vi "Licor data processing.vi"(8 "command parameter":T2={"CO2 ref"=392.0, "CO2 span"=372.0, "H2O ref"=0.0, "H2O span"=0.0, "Zi"=0.0, "Zt"=1.2, "Zm"=0.0, "S"=0.0, "Temp [C]"=50.0, "Pressure [hPa]"=135.0, "Licor-Sources"=["CO2A W", "CO2B W", "H2OA W", "H2OB W", "T C", "T V", "P kPa", "P V", "RH %", "CO2A um/m", "CO2B um/m", "H2OA mm/m", "H2OB mm/m"], "Licor-Pump"="Off", "Zeitstempel"=timestamp(0 s since 1904-01-01)} {"Pressure [hPa]" format="%_5g"; "Temp [C]" format="%.2f"; "CO2 ref" format="%.2f"; "CO2 span" format="%.2g"; "H2O ref" format="%.2g"; "H2O span" format="%.2g"; "Zt" format="%#_4g"}, 9 "mittel CO2B W":dbl[](array[numeric]), 10 "mittel CO2A W":dbl[](array[numeric]), 11 "data":T1[](array[typedef]) {"time (global)" format="%<%H:%M:%S\n%d/%m/%Y>T"}) -> (0 "time; CO2 data":dbl[][](array[numeric]), 1 "mittel CO2B W out":dbl[](array[numeric]), 2 "mittel CO2A W out":dbl[](array[numeric]), 3 "command parameter":T2={"CO2 ref"=0.0, "CO2 span"=0.0, "H2O ref"=0.0, "H2O span"=0.0, "Zi"=0.0, "Zt"=0.0, "Zm"=0.0, "S"=0.0, "Temp [C]"=50.0, "Pressure [hPa]"=135.0, "Licor-Sources"=["CO2A W", "CO2B W", "H2OA W", "H2OB W", "T C", "T V", "P kPa", "P V", "RH %", "CO2A um/m", "CO2B um/m", "H2OA mm/m", "H2OB mm/m"], "Licor-Pump"="Off", "Zeitstempel"=timestamp(0 s since 1904-01-01)} {"Pressure [hPa]" format="%_5g"; "Temp [C]" format="%.2f"; "CO2 ref" format="%.2f"; "CO2 span" format="%.2g"; "H2O ref" format="%.2g"; "H2O span" format="%.2g"; "Zt" format="%#_4g"})   [LabVIEW 2017, in "Licor-Steuerung.lvlib"]
uses:
  Licor-Steuerung.lvlib
  control/Licor-Parameter.ctl
  LicorLI7000/conventions/Licor-Source.ctl
  control/Licor-Pump.ctl
  LicorLI7000/conventions/output line.ctl
  LicorLI7000/Z parameter.ctl
  LicorLI7000/LicorLI7000.lvlib
panel:
  in  "get Source":string(combo)="CO2A W"
  out "calibration data out":dbl[][](array[numeric])
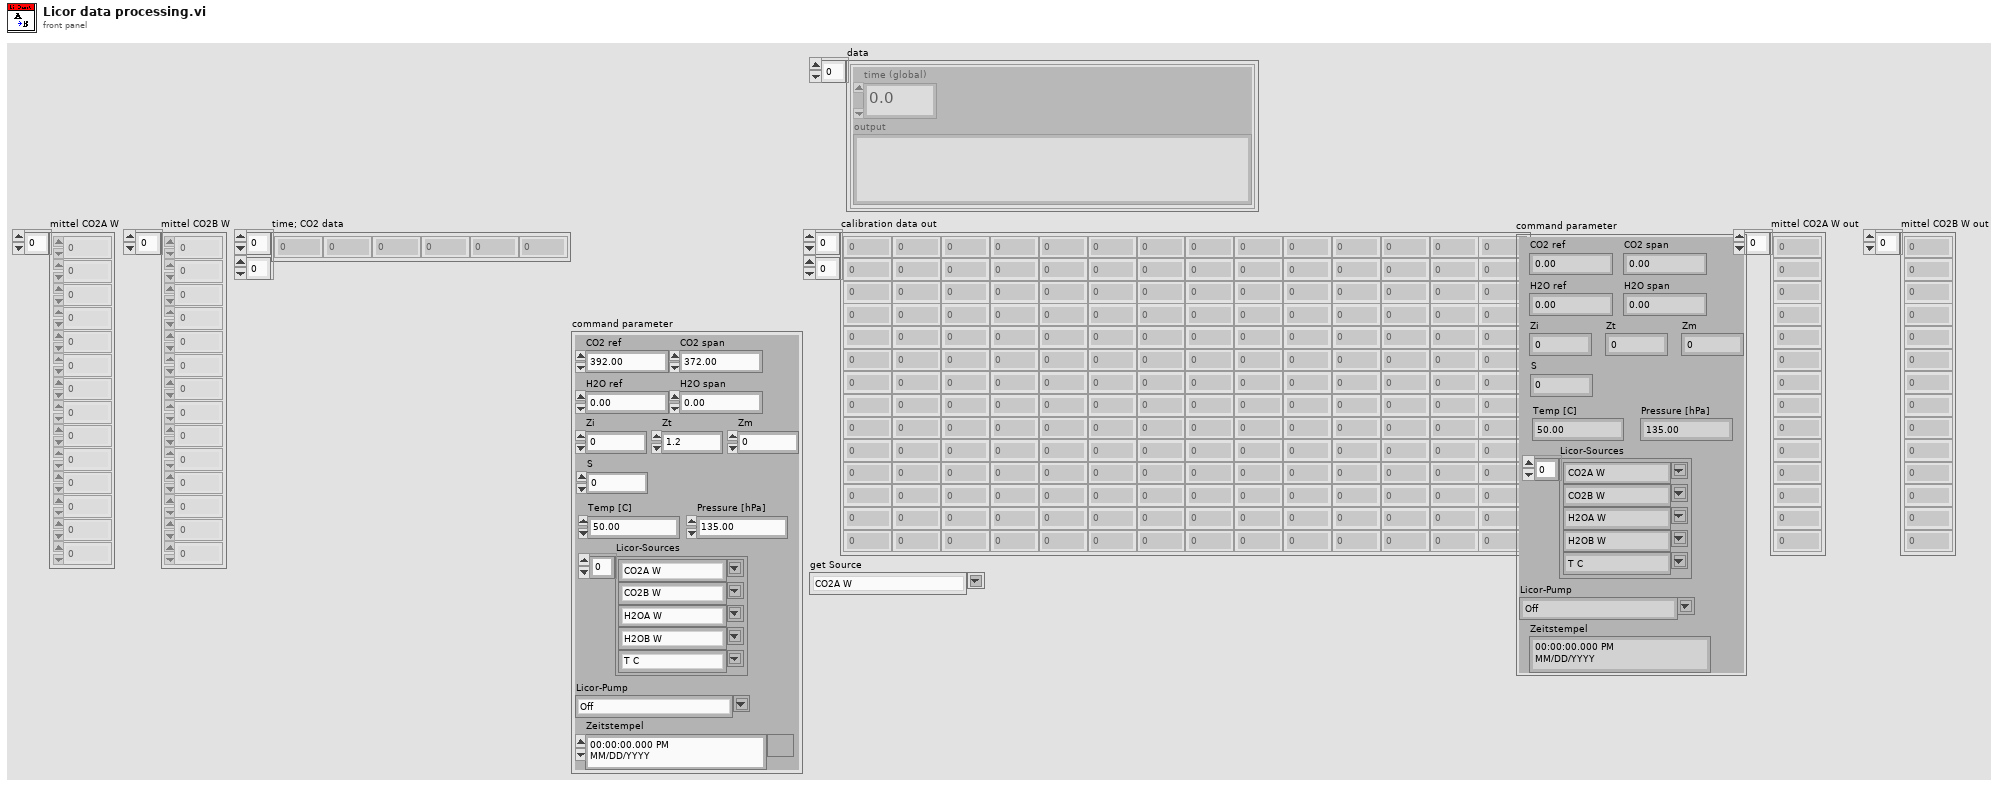
[diagram p1: front panel]
types:
  T1 = typedef "LicorLI7000.lvlib/output line.ctl" = cluster{"time (global)":dbl, "output":string}
  T2 = typedef "Licor-Steuerung.lvlib/Licor-Parameter.ctl" = cluster{"CO2 ref":dbl, "CO2 span":dbl, "H2O ref":dbl, "H2O span":dbl, "Zi":dbl, "Zt":dbl, "Zm":dbl, "S":dbl, "Temp [C]":dbl, "Pressure [hPa]":dbl, "Licor-Sources":T3[], "Licor-Pump":T4, "Zeitstempel":timestamp}
  T3 = typedef "LicorLI7000.lvlib/Licor-Source.ctl" = string
  T4 = typedef "Licor-Steuerung.lvlib/Licor-Pump.ctl" = string
  T5 = typedef "LicorLI7000.lvlib/Z parameter.ctl" = cluster{"zi":dbl, "zt":dbl, "zm":dbl}
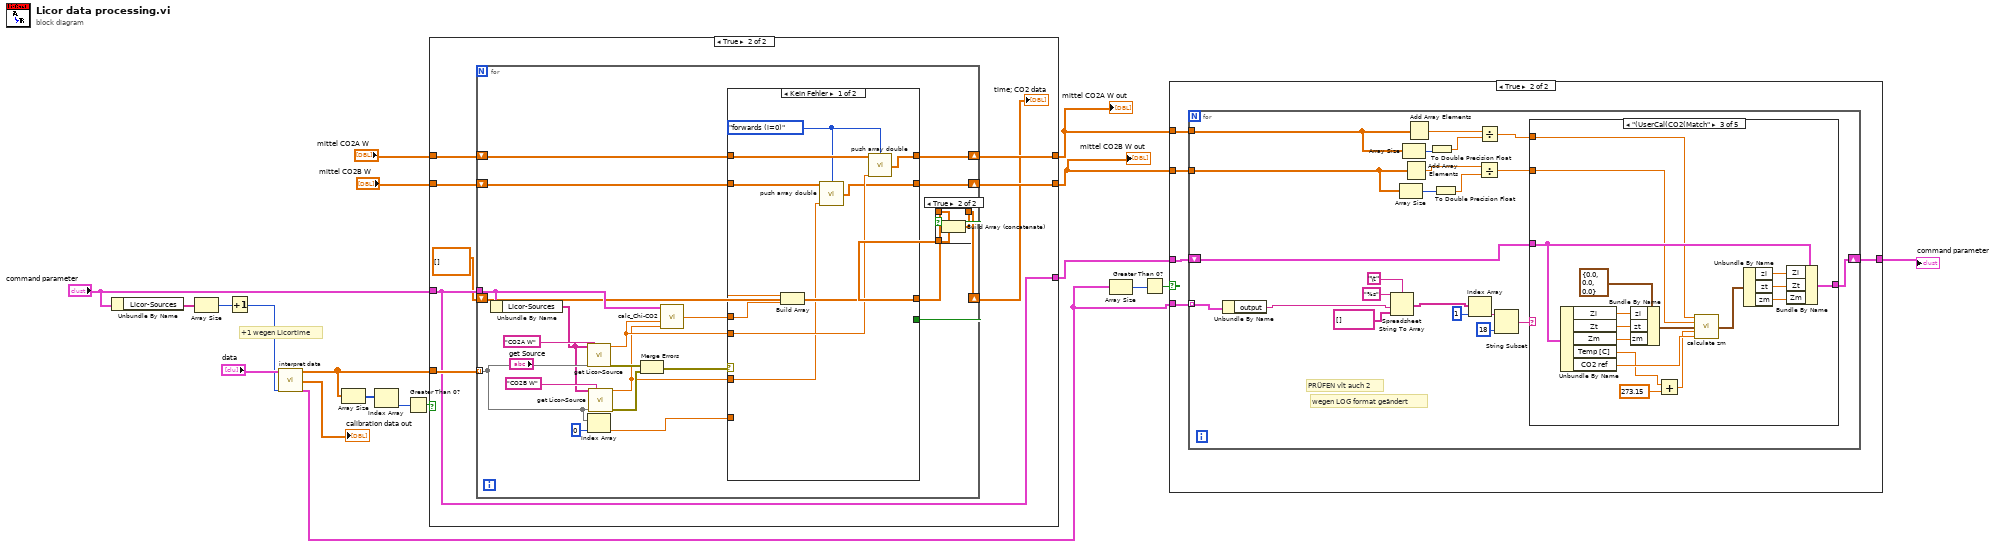
[diagram p0: block diagram]
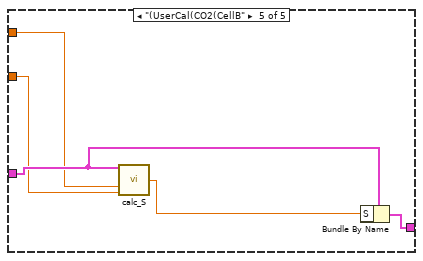
[diagram p6: hidden frame]
diagram:
  # "+1 wegen Licortime"
  n1 = Unbundle By Name("command parameter") -> ("Licor-Sources"=w4:T3[])
  n2 = Array Size(array=w4) -> (size(s)=w3:i32)
  n3 = Increment(x=w3) -> (x+1=w2:i32)
  n4 = call "interpret data.vi"("data"="data", "anzahl sources"=w2) -> ("source data out"=w18:dbl[][], "calibration data out"=→"calibration data out":dbl[][], "log"=w1:T1[])  [unwired: 11 in]
  n5 = Array Size(array=w18) -> (size(s)=w17:i32[])
  n6 = Index Array(array=w17) -> (element=w16:i32)  [unwired: 1 in]
  n7 = Greater Than 0?(x=w16) -> (x > 0?=w19:bool)
  n8 = case shown="True" w19 {
    tunnel: w18 -> [_ w30]
    tunnel: "command parameter" -> [w22 w29]
    tunnel: [w22 w29] -> w14
    tunnel: "mittel CO2A W" -> [w21 w28]
    tunnel: "mittel CO2B W" -> [w20 w27]
    tunnel: [w21 w26] -> w10
    tunnel: [w20 w25] -> w9
    frame False {
    }
    frame True {
      n9 = for {
        tunnel: w30 -> [w38] mode=indexing
        tunnel: w29 -> [w34]
        shift-right: [w41] -> w26
        shift-left: w28 -> [w43]
        shift-right: [w40] -> w25
        shift-left: w27 -> [w42]
        shift-right: [w31] -> w24
        shift-left: dbl[][] [] ("Array") -> [w32]
        n10 = Unbundle By Name(w34) -> ("Licor-Sources"=w33:T3[])
        n11 = call "get Licor-Source.vi"("Sources"=w33, "get Source"="CO2A W", "source data"=w38) -> ("value"=w45:dbl, "Fehlerkonstante"=w48:errorcluster)  [unwired: 10 in, 1 out]
        n12 = Index Array(array=w38, index=0 ("Index")) -> (element=w37:dbl)
        n13 = call "get Licor-Source.vi"("Sources"=w33, "get Source"="CO2B W", "source data"=w38) -> ("value"=w44:dbl, "Fehlerkonstante"=w49:errorcluster)  [unwired: 10 in, 1 out]
        n14 = Merge Errors(w48, w49) -> (w47:errorcluster)
        n15 = call "calc_Chi-CO2.vi"("command parameter"=w34, "Raw_CO2_A"=w45, "Raw_CO2_B"=w44) -> ("Chi_CO2_B"=w46:dbl)  [unwired: 12 in]
        n16 = case shown="Kein Fehler" w47 {
          tunnel: [w57 dbl[] []] -> w36
          tunnel: w46 -> [w66 _]
          tunnel: w44 -> [w59 _]
          tunnel: w45 -> [w64 _]
          tunnel: w43 -> [w65 w70]
          tunnel: w42 -> [w62 w69]
          tunnel: [w63 w70] -> w41
          tunnel: [w60 w69] -> w40
          tunnel: w37 -> [w58 _]
          tunnel: [TRUE FALSE] -> w35
          frame No Error {
            w61 = enum16{"forwards (i=0)", "backwards (i=n)"}."forwards (i=0)" ("mode")
            n17 = Build Array(w58, w66) -> (w57:dbl[])
            n18 = call "push array double.vi"("Array"=w62, "mode"=w61, "Element"=w59) -> ("Array out"=w60:dbl[])  [unwired: 12 in]
            n19 = call "push array double.vi"("Array"=w65, "mode"=w61, "Element"=w64) -> ("Array out"=w63:dbl[])  [unwired: 12 in]
          }
          frame Error {
          }
        }
        n20 = case shown="True" w35 {
          tunnel: w32 -> [w52 w54]
          tunnel: w36 -> [_ w53]
          tunnel: [w52 w55] -> w31
          frame False {
          }
          frame True {
            n21 = Build Array (concatenate)(w54, w53) -> (w55:dbl[][])
          }
        }
      }
      "time; CO2 data" <- w24
    }
  }
  "mittel CO2A W out" <- w10
  "mittel CO2B W out" <- w9
  n22 = Array Size(array=w1) -> (size(s)=w6:i32)
  n23 = Greater Than 0?(x=w6) -> (x > 0?=w13:bool)
  n24 = case shown="True" w13 {
    tunnel: w1 -> [_ w76]
    tunnel: w14 -> [w71 w75]
    tunnel: w9 -> [_ w74]
    tunnel: w10 -> [_ w73]
    tunnel: [w71 w72] -> w8
    frame False {
    }
    frame True {
      n25 = for {
        tunnel: w76 -> [w78] mode=indexing
        shift-right: [w95] -> w72
        shift-left: w75 -> [w83]
        tunnel: w73 -> [w85]
        tunnel: w74 -> [w84]
        # "wegen LOG format geändert"
        # "PRÜFEN vlt auch 2"
        n26 = Unbundle By Name(w78) -> ("output"=w77:string)
        n27 = Spreadsheet String To Array(delimiter (Tab)="\t", format string="%s", spreadsheet string=w77, array type (2D Dbl)=string[] []) -> (array=w79:string[])
        n28 = Array Size(array=w84) -> (size(s)=w92:i32)
        n29 = Array Size(array=w85) -> (size(s)=w91:i32)
        n30 = Add Array Elements(numeric array=w84) -> (sum=w89:dbl)
        n31 = Add Array Elements(numeric array=w85) -> (sum=w93:dbl)
        n32 = To Double Precision Float(number=w91) -> (double precision float=w90:dbl)
        n33 = To Double Precision Float(number=w92) -> (double precision float=w88:dbl)
        n34 = Index Array(array=w79, index=1 ("Index")) -> (element=w96:string)
        n35 = Divide(x=w89, y=w88) -> (x/y=w86:dbl)
        n36 = Divide(x=w93, y=w90) -> (x/y=w87:dbl)
        n37 = String Subset(string=w96, length (rest)=18 ("Länge (Rest)")) -> (substring=w94:string)  [unwired: 1 in]
        n38 = case shown="\"(UserCal(CO2(Match\"" w94 {
          tunnel: w83 -> [w99 w100 w115 w118 w123]
          tunnel: [w99 w100 w117 w118 w122] -> w95
          tunnel: w87 -> [_ _ w110 _ w120]
          tunnel: w86 -> [_ _ w109 _ w119]
          frame "False", Default {
          }
          frame "(UserCal(H2O(Match" {
          }
          frame "(UserCal(CO2(Match" {
            n39 = Unbundle By Name(w115) -> ("Zi"=w114:dbl, "Zt"=w113:dbl, "Zm"=w112:dbl, "Temp [C]"=w102:dbl, "CO2 ref"=w108:dbl)
            n40 = Bundle By Name(cluster=T5 {"zi"=0.0, "zt"=0.0, "zm"=0.0} ("Z"), "zi"=w114, "zt"=w113, "zm"=w112) -> (w111:T5)
            n41 = Add(x=w102, y=273.15) -> (x+y=w101:dbl)
            n42 = call "calculate zm.vi"("W_A [raw signal]"=w110, "W_B [raw signal]"=w109, "Z"=w111, "T [K]"=w101, "Chi_A"=w108) -> ("Z (out)"=w107:T5)  [unwired: 10 in]
            n43 = Unbundle By Name(w107) -> ("zi"=w106:dbl, "zt"=w105:dbl, "zm"=w104:dbl)
            n44 = Bundle By Name(cluster=w115, "Zi"=w106, "Zt"=w105, "Zm"=w104) -> (w117:T2)
          }
          frame "(UserCal(H2O(CellB" {
          }
          frame "(UserCal(CO2(CellB" {
            n45 = call "calc_S.vi"("command parameter"=w123, "Chi_CO2_A"=w120, "Chi_CO2_B"=w119) -> ("S"=w121:dbl)  [unwired: 12 in]
            n46 = Bundle By Name(cluster=w123, "S"=w121) -> (w122:T2)
          }
        }
      }
    }
  }
  "command parameter" <- w8
